vi "OpenFileDAQ.vi"(0 "DAQ File Name":string, 3 "error in":errorcluster) -> (7 "appended path":path, 8 "t0":timestamp, 10 "error out":errorcluster)   [LabVIEW 2019, in "DAQ.lvclass"]
uses:
  DAQ.lvclass
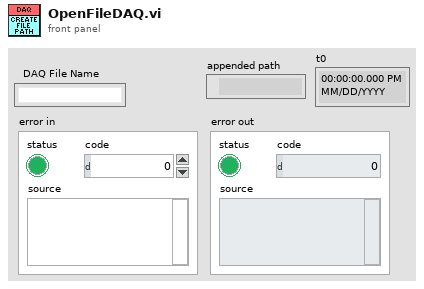
[diagram p1: front panel]
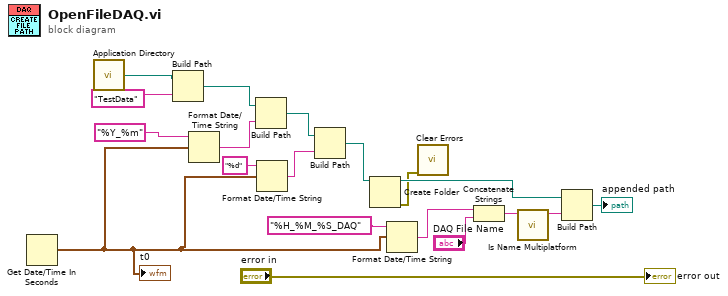
[diagram p0: block diagram]
diagram:
  n1 = Get Date/Time In Seconds() -> (seconds since 1Jan1904=w1:timestamp)
  "t0" <- w1
  n2 = call <vilib>:"Application Directory.vi"() -> ("Application Directory"=w16:path)
  n3 = Build Path(base path=w16, name or relative path="TestData") -> (appended path=w6:path)
  n4 = Format Date/Time String(time format string (%c)="%Y_%m", seconds (now)=w1) -> (date/time string=w7:string)  [unwired: 1 in]
  n5 = Build Path(base path=w6, name or relative path=w7) -> (appended path=w5:path)
  n6 = Format Date/Time String(time format string (%c)="%d", seconds (now)=w1) -> (date/time string=w3:string)  [unwired: 1 in]
  n7 = Build Path(base path=w5, name or relative path=w3) -> (appended path=w2:path)
  n8 = Create Folder(path (use dialog)=w2) -> (created path=w12:path, error out=w11:errorcluster)  [unwired: 2 in, 1 out]
  n9 = Format Date/Time String(time format string (%c)="%H_%M_%S_DAQ", seconds (now)=w1) -> (date/time string=w18:string)  [unwired: 1 in]
  n10 = call <vilib>:"Clear Errors.vi"("error in (no error)"=w11) -> ()  [unwired: 5 in, 2 out]
  n11 = Concatenate Strings(w18, "DAQ File Name") -> (w14:string)
  n12 = call <vilib>:"Is Name Multiplatform.vi"("filename"=w14) -> ("suggested filename"=w13:string)  [unwired: 6 in, 4 out]
  n13 = Build Path(base path=w12, name or relative path=w13) -> (appended path=→"appended path":path)
  "error out" <- "error in"
